vi "Begin.vi"() -> (0 "error out":errorcluster)   [LabVIEW 2013]
doc: "Called before other user functions, this VI is expected to open initial I/O refnums, load in file data, and do all program initialization. Notice that the <B>error out</B> terminal is simply used for data flow. Wiring it to other structures or subVIs ensures that this VI runs first."
uses:
  <vilib>/Rock Robotics/WPI/DriverStation/WPI_DriverStationRobotMode2.ctl
  <vilib>/Rock Robotics/WPI/Joystick/WPI_JoystickDeviceEnum.ctl
  <vilib>/Rock Robotics/SystemInterfaces/DIO/FPGA_DIOPWMChannel.ctl
  <vilib>/Rock Robotics/SystemInterfaces/AI/FPGA_AIChannel.ctl
  <vilib>/Rock Robotics/SystemInterfaces/DIO/FPGA_DIOChannel.ctl
  <vilib>/Rock Robotics/WPI/Encoder/WPI_EncoderType.ctl
  Robot Global Data.vi
  <vilib>/Rock Robotics/WPI/MotorControl/WPI_MotorControlOpen Talon.vi
  <vilib>/Rock Robotics/WPI/Counter/WPI_CounterDigitalInputToDigitalSource.vi
  <vilib>/Utility/file.llb/Read From Spreadsheet File (DBL).vi
  Globals/Auto.vi
  Globals/Homes.vi
  <vilib>/Rock Robotics/WPI/Camera/WPI_CameraWhite Balance Values.ctl
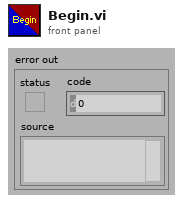
[diagram p1: front panel]
types:
  T1 = typedef "FPGA_DIOPWMChannel.ctl" = enum8{"PWM 1", "PWM 2", "PWM 3", "PWM 4", "PWM 5", "PWM 6", "PWM 7", "PWM 8", "PWM 9", "PWM 10", "Invalid"}
  T2 = typedef "FPGA_AIChannel.ctl" = enum8{"AI 1", "AI 2", "AI 3", "AI 4", "AI 5", "AI 6", "AI 7", "AI 8", "Invalid"}
  T3 = typedef "FPGA_DIOChannel.ctl" = enum8{"DIO 1", "DIO 2", "DIO 3", "DIO 4", "DIO 5", "DIO 6", "DIO 7", "DIO 8", "DIO 9", "DIO 10", "DIO 11", "DIO 12", "DIO 13", "DIO 14", "Invalid"}
  T4 = typedef "WPI_EncoderType.ctl" = enum16{"1x", "2x", "4x"}
  T5 = typedef "WPI_JoystickDeviceEnum.ctl" = enum16{"USB 1", "USB 2", "USB 3", "USB 4", "Kinect 1", "Kinect 2"}
  T6 = typedef "WPI_DriverStationRobotMode2.ctl" = enum16{"Autonomous Disabled", "Autonomous Enabled", "Teleop Disabled", "Teleop Enabled", "Timeout", "Finish", "Test Disabled", "Test Enabled"}
  T7 = typedef "WPI_JoystickDevRef.ctl" = cluster{"Device":T5}
  T8 = typedef "WPI_MotorControlDeviceRef.ctl" = cluster{"DeviceStatus":errorcluster, "Type":enum16{"PWM", "CAN"}, "PWM":cluster{"Digital Module":T9, "PWM Channel":T1, "DeadBand":T10}, "CAN":cluster{"Device Number":u8, "Control Mode":T11, "Semaphore":T12, "Max Vout":dbl}, "Invert":bool, "TransformRef":T13, "InvTransformRef":T13}
  T9 = typedef "FPGA_TypedefDigitalModule.ctl" = enum16{"Digital Module 1", "Digital Module 2"}
  T10 = typedef "WPI_PWMDeadband.ctl" = cluster{"Name":string, "maxPositivePwm":i32, "minPositivePwm":i32, "centerPwm":i32, "maxNegativePwm":i32, "minNegativePwm":i32, "angularRange":u16}
  T11 = typedef "WPI_CANJaguar_ControlMode.ctl" = enum8{"Percent VBus", "Current", "Speed", "Position", "Voltage"}
  T12 = typedef "Semaphore RefNum" = refnum<k1>
  T13 = typedef "WPI_PWMTransform_ConPane.ctl" = refnum<vi>
  T14 = typedef "WPI_CameraWhite Balance Values.ctl" = enum16{"Auto", "Fixed indoor", "Fixed outdoor 1", "Fixed outdoor 2", "Fixed fluorescent 1", "Fixed fluorescent 2", "Hold current"}
  T15 = typedef "WPI_CameraDevRef.ctl" = cluster{"Camera Address":string, "CameraStatus":errorcluster, "Acquire Image Notifier":refnum<notifier>}
  T16 = typedef "WPI_AnalogChannelDevRef.ctl" = cluster{"DevStatus":errorcluster, "Analog Module":T17, "Analog Channel":T2}
  T17 = typedef "FPGA_TypedefAnalogModule.ctl" = enum16{"Analog Module 1", "Analog Module 2"}
  T18 = typedef "WPI_DigitalInputDevRef.ctl" = cluster{"DevStatus":errorcluster, "DIO Channel":T3, "Digital Module":T9}
  T19 = typedef "FPGA_CounterEncoderSourceConvertionLVSourceType.ctl" = cluster{"DevStatus":errorcluster, "AnalogTriggerMode?":bool, "DigitalMode":cluster{"Digital Module":T9, "DIO Channel":T20}, "AnalogTriggerMode":cluster{"AnalogTriggerIndex":T21, "OutputType":T22}}
  T20 = typedef "FPGA_DIODigitalSourceChannel.ctl" = enum8{"DIO 1", "DIO 2", "DIO 3", "DIO 4", "DIO 5", "DIO 6", "DIO 7", "DIO 8", "DIO 9", "DIO 10", "DIO 11", "DIO 12", "DIO 13", "DIO 14", "Disabled"}
  T21 = typedef "FPGA_AnalogTriggerIndex.ctl" = enum8{"Trig 0", "Trig 1", "Trig 2", "Trig 3", "Trig 4", "Trig 5", "Trig 6", "Trig 7", "Invalid"}
  T22 = typedef "FPGA_AnalogTriggerOutType.ctl" = enum16{"InWindow", "TriggerState", "Rising", "Falling"}
  T23 = typedef "WPI_EncoderDevRef.ctl" = cluster{"DevStatus":errorcluster, "EncoderIndex":T24, "CounterIndex":T25, "DistancePerCount":dbl, "Decoding Type":T4}
  T24 = typedef "FPGA_EncoderIdx.ctl" = enum8{"Enc 0", "Enc 1", "Enc 2", "Enc 3", "Invalid"}
  T25 = typedef "FPGA_CounterCtrSystemIndex.ctl" = enum8{"Ctr 0", "Ctr 1", "Ctr 2", "Ctr 3", "Ctr 4", "Ctr 5", "Ctr 6", "Ctr 7", "Invalid"}
  T26 = typedef "WPI_DigitalOutputDevRef.ctl" = cluster{"Digital Module":T9, "DIO Channel":T3, "DevStatus":errorcluster}
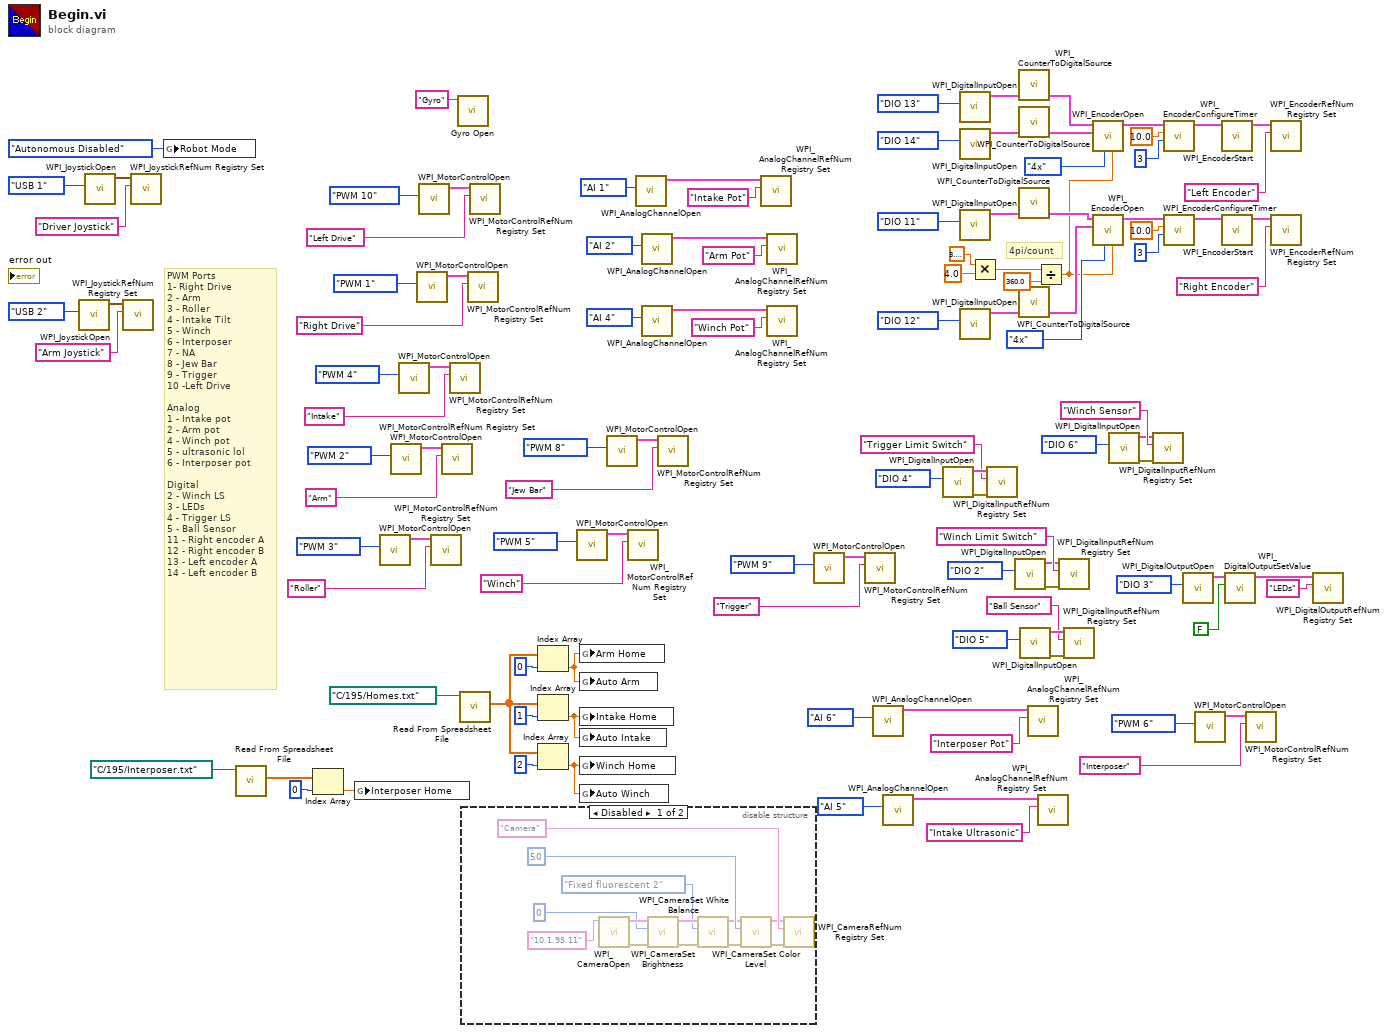
[diagram p0: block diagram]
diagram:
  # "4pi/count"
  # "PWM Ports\n1- Right Drive\n2 - Arm\n3 - Roller\n4 - Intake Tilt \n5 - Winch\n6 - Interposer \n7 - NA\n8 - Jew Bar\n9 - Trigger\n10 -Left Drive\n\nAnalog\n1 - Intake pot\n2 - Arm pot\n4 - Winch pot\n5 - ultrasonic lol\n6 - Interposer pot\n\nDigital \n2 - Winch LS\n3 - LEDs\n4 - Trigger LS\n5 - Ball Sensor\n11 - Right encoder A\n12 - Right encoder B\n13 - Left encoder A\n14 - Left encoder B"
  n1 = call <vilib>:"WPI_JoystickOpen.vi"("JoystickDevice"=WPI_JoystickDeviceEnum."USB 2") -> ("JoystickDevRef"=w109:T7)  [unwired: 10 in]
  n2 = call <vilib>:"WPI_JoystickOpen.vi"("JoystickDevice"=WPI_JoystickDeviceEnum."USB 1") -> ("JoystickDevRef"=w112:T7)  [unwired: 10 in]
  n3 = call <vilib>:"WPI_JoystickRefNum Registry Set.vi"("refnum name"="Arm Joystick", "JoystickDevRef"=w109) -> ()  [unwired: 8 in, 2 out]
  n4 = call <vilib>:"WPI_JoystickRefNum Registry Set.vi"("refnum name"="Driver Joystick", "JoystickDevRef"=w112) -> ()  [unwired: 8 in, 2 out]
  n5 = global write "Robot Global Data.vi" "Robot Mode"(WPI_DriverStationRobotMode2."Autonomous Disabled" ("Robot Mode")) -> ()
  n6 = call-poly <vilib>:"Read From Spreadsheet File.vi"("file path (dialog if empty)"=path "C:/195/Interposer.txt" ("file path (use dialog)")) -> ("first row"=w2:dbl[])  [unwired: 6 in, 4 out]
  n7 = Index Array(array=w2, index=0) -> (element=w1:dbl)
  n8 = global write "Homes.vi" "Interposer Home"(w1) -> ()
  n9 = call-poly <vilib>:"WPI_MotorControlOpen.vi"("PWM Channel"=FPGA_DIOPWMChannel."PWM 3") -> ("MotorControlDeviceRef"=w95:T8)  [unwired: 9 in, 1 out]
  n10 = call-poly <vilib>:"WPI_MotorControlOpen.vi"("PWM Channel"=FPGA_DIOPWMChannel."PWM 2") -> ("MotorControlDeviceRef"=w98:T8)  [unwired: 9 in, 1 out]
  n11 = call-poly <vilib>:"WPI_MotorControlOpen.vi"("PWM Channel"=FPGA_DIOPWMChannel."PWM 4") -> ("MotorControlDeviceRef"=w99:T8)  [unwired: 9 in, 1 out]
  n12 = call-poly <vilib>:"WPI_MotorControlOpen.vi"("PWM Channel"=FPGA_DIOPWMChannel."PWM 1") -> ("MotorControlDeviceRef"=w102:T8)  [unwired: 9 in, 1 out]
  n13 = call-poly <vilib>:"WPI_MotorControlOpen.vi"("PWM Channel"=FPGA_DIOPWMChannel."PWM 10") -> ("MotorControlDeviceRef"=w107:T8)  [unwired: 9 in, 1 out]
  n14 = call <vilib>:"WPI_MotorControlRefNum Registry Set.vi"("refnum name"="Roller", "MotorControlDevRef"=w95) -> ()  [unwired: 8 in, 2 out]
  n15 = call <vilib>:"WPI_MotorControlRefNum Registry Set.vi"("refnum name"="Arm", "MotorControlDevRef"=w98) -> ()  [unwired: 8 in, 2 out]
  n16 = call <vilib>:"WPI_MotorControlRefNum Registry Set.vi"("refnum name"="Intake", "MotorControlDevRef"=w99) -> ()  [unwired: 8 in, 2 out]
  n17 = call "Gyro Open.vi"("refnum name"="Gyro") -> ()  [unwired: 10 in, 1 out]
  n18 = call-poly <vilib>:"Read From Spreadsheet File.vi"("file path (dialog if empty)"=path "C:/195/Homes.txt" ("file path (use dialog)")) -> ("first row"=w28:dbl[])  [unwired: 6 in, 4 out]
  n19 = disable-structure shown="Disabled" {
    frame Disabled {
      n20 = call <vilib>:"WPI_CameraOpen.vi"("Camera Address"="10.1.95.11") -> ("error out"=w121:errorcluster, "CameraDevRef"=w126:T15)  [unwired: 1 in, 8 out]
      n21 = call <vilib>:"WPI_CameraSet Brightness.vi"("error in (no error)"=w121, "Brightness"=0, "CameraDevRef"=w126) -> ("error out"=w122:errorcluster, "CameraDevRef Out"=w125:T15)  [unwired: 7 in]
      n22 = call <vilib>:"WPI_CameraSet White Balance.vi"("error in (no error)"=w122, "White Balance"=WPI_CameraWhite_Balance_Values."Fixed fluorescent 2", "CameraDevRef"=w125) -> ("error out"=w117:errorcluster, "CameraDevRef Out"=w115:T15)  [unwired: 7 in]
      n23 = call <vilib>:"WPI_CameraSet Color Level.vi"("error in (no error)"=w117, "Color Level"=50, "CameraDevRef"=w115) -> ("error out"=w118:errorcluster, "CameraDevRef Out"=w119:T15)  [unwired: 7 in]
      n24 = call <vilib>:"WPI_CameraRefNum Registry Set.vi"("error in (no error)"=w118, "refnum name"="Camera", "CameraDevRef"=w119) -> ()  [unwired: 9 out]
    }
    frame Enabled {
    }
  }
  n25 = call <vilib>:"WPI_MotorControlRefNum Registry Set.vi"("refnum name"="Right Drive", "MotorControlDevRef"=w102) -> ()  [unwired: 8 in, 2 out]
  n26 = call <vilib>:"WPI_MotorControlRefNum Registry Set.vi"("refnum name"="Left Drive", "MotorControlDevRef"=w107) -> ()  [unwired: 8 in, 2 out]
  n27 = Index Array(array=w28, index=0) -> (element=w17:dbl)
  n28 = Index Array(array=w28, index=1) -> (element=w15:dbl)
  n29 = Index Array(array=w28, index=2) -> (element=w16:dbl)
  n30 = call-poly <vilib>:"WPI_MotorControlOpen.vi"("PWM Channel"=FPGA_DIOPWMChannel."PWM 5") -> ("MotorControlDeviceRef"=w81:T8)  [unwired: 9 in, 1 out]
  n31 = global write "Homes.vi" "Arm Home"(w17) -> ()
  n32 = global write "Auto.vi" "Auto Arm"(w17) -> ()
  n33 = global write "Homes.vi" "Intake Home"(w15) -> ()
  n34 = global write "Auto.vi" "Auto Intake"(w15) -> ()
  n35 = global write "Homes.vi" "Winch Home"(w16) -> ()
  n36 = global write "Auto.vi" "Auto Winch"(w16) -> ()
  n37 = call-poly <vilib>:"WPI_MotorControlOpen.vi"("PWM Channel"=FPGA_DIOPWMChannel."PWM 8") -> ("MotorControlDeviceRef"=w76:T8)  [unwired: 9 in, 1 out]
  n38 = call <vilib>:"WPI_MotorControlRefNum Registry Set.vi"("refnum name"="Winch", "MotorControlDevRef"=w81) -> ()  [unwired: 8 in, 2 out]
  n39 = call <vilib>:"WPI_AnalogChannelOpen.vi"("Analog Channel"=FPGA_AIChannel."AI 1") -> ("AIDeviceRef"=w92:T16)  [unwired: 9 in, 1 out]
  n40 = call <vilib>:"WPI_AnalogChannelOpen.vi"("Analog Channel"=FPGA_AIChannel."AI 2") -> ("AIDeviceRef"=w87:T16)  [unwired: 9 in, 1 out]
  n41 = call <vilib>:"WPI_AnalogChannelOpen.vi"("Analog Channel"=FPGA_AIChannel."AI 4") -> ("AIDeviceRef"=w86:T16)  [unwired: 9 in, 1 out]
  n42 = call <vilib>:"WPI_MotorControlRefNum Registry Set.vi"("refnum name"="Jew Bar", "MotorControlDevRef"=w76) -> ()  [unwired: 8 in, 2 out]
  n43 = call <vilib>:"WPI_AnalogChannelRefNum Registry Set.vi"("refnum name"="Intake Pot", "AIDeviceRef"=w92) -> ()  [unwired: 8 in, 2 out]
  n44 = call <vilib>:"WPI_AnalogChannelRefNum Registry Set.vi"("refnum name"="Arm Pot", "AIDeviceRef"=w87) -> ()  [unwired: 8 in, 2 out]
  n45 = call <vilib>:"WPI_AnalogChannelRefNum Registry Set.vi"("refnum name"="Winch Pot", "AIDeviceRef"=w86) -> ()  [unwired: 8 in, 2 out]
  n46 = call-poly <vilib>:"WPI_MotorControlOpen.vi"("PWM Channel"=FPGA_DIOPWMChannel."PWM 9") -> ("MotorControlDeviceRef"=w71:T8)  [unwired: 9 in, 1 out]
  n47 = call <vilib>:"WPI_MotorControlRefNum Registry Set.vi"("refnum name"="Trigger", "MotorControlDevRef"=w71) -> ()  [unwired: 8 in, 2 out]
  n48 = call <vilib>:"WPI_AnalogChannelOpen.vi"("Analog Channel"=FPGA_AIChannel."AI 6") -> ("AIDeviceRef"=w8:T16)  [unwired: 9 in, 1 out]
  n49 = call <vilib>:"WPI_AnalogChannelOpen.vi"("Analog Channel"=FPGA_AIChannel."AI 5") -> ("AIDeviceRef"=w27:T16)  [unwired: 9 in, 1 out]
  n50 = call <vilib>:"WPI_DigitalInputOpen.vi"("DIO Channel"=FPGA_DIOChannel."DIO 4") -> ("error out"=w79:errorcluster, "DigitalInputDevRef"=w78:T18)  [unwired: 9 in]
  n51 = call <vilib>:"WPI_DigitalInputOpen.vi"("DIO Channel"=FPGA_DIOChannel."DIO 13") -> ("DigitalInputDevRef"=w47:T18)  [unwired: 9 in, 1 out]
  n52 = call <vilib>:"WPI_DigitalInputOpen.vi"("DIO Channel"=FPGA_DIOChannel."DIO 14") -> ("DigitalInputDevRef"=w46:T18)  [unwired: 9 in, 1 out]
  n53 = call <vilib>:"WPI_DigitalInputOpen.vi"("DIO Channel"=FPGA_DIOChannel."DIO 11") -> ("DigitalInputDevRef"=w45:T18)  [unwired: 9 in, 1 out]
  n54 = call <vilib>:"WPI_DigitalInputOpen.vi"("DIO Channel"=FPGA_DIOChannel."DIO 12") -> ("DigitalInputDevRef"=w44:T18)  [unwired: 9 in, 1 out]
  n55 = Multiply(x=3.141592653589793, y=4.0) -> (x*y=w37:dbl)
  n56 = call <vilib>:"WPI_DigitalInputRefNum Registry Set.vi"("error in (no error)"=w79, "refnum name"="Trigger Limit Switch", "DigitalInputDevRef"=w78) -> ()  [unwired: 7 in, 2 out]
  n57 = call <vilib>:"WPI_DigitalInputOpen.vi"("DIO Channel"=FPGA_DIOChannel."DIO 2") -> ("error out"=w67:errorcluster, "DigitalInputDevRef"=w68:T18)  [unwired: 9 in]
  n58 = call-poly <vilib>:"WPI_CounterToDigitalSource.vi"("DigitalInputDevRef"=w47) -> ("Digital Source"=w58:T19)  [unwired: 6 in]
  n59 = call-poly <vilib>:"WPI_CounterToDigitalSource.vi"("DigitalInputDevRef"=w46) -> ("Digital Source"=w57:T19)  [unwired: 6 in]
  n60 = call-poly <vilib>:"WPI_CounterToDigitalSource.vi"("DigitalInputDevRef"=w45) -> ("Digital Source"=w55:T19)  [unwired: 6 in]
  n61 = call-poly <vilib>:"WPI_CounterToDigitalSource.vi"("DigitalInputDevRef"=w44) -> ("Digital Source"=w56:T19)  [unwired: 6 in]
  n62 = call <vilib>:"WPI_DigitalInputOpen.vi"("DIO Channel"=FPGA_DIOChannel."DIO 5") -> ("error out"=w20:errorcluster, "DigitalInputDevRef"=w19:T18)  [unwired: 9 in]
  n63 = call <vilib>:"WPI_AnalogChannelRefNum Registry Set.vi"("refnum name"="Interposer Pot", "AIDeviceRef"=w8) -> ()  [unwired: 8 in, 2 out]
  n64 = Divide(x=w37, y=360.0) -> (x/y=w35:dbl)
  n65 = call <vilib>:"WPI_AnalogChannelRefNum Registry Set.vi"("refnum name"="Intake Ultrasonic", "AIDeviceRef"=w27) -> ()  [unwired: 8 in, 2 out]
  n66 = call <vilib>:"WPI_DigitalInputRefNum Registry Set.vi"("error in (no error)"=w67, "refnum name"="Winch Limit Switch", "DigitalInputDevRef"=w68) -> ()  [unwired: 7 in, 2 out]
  n67 = call <vilib>:"WPI_DigitalInputRefNum Registry Set.vi"("error in (no error)"=w20, "refnum name"="Ball Sensor", "DigitalInputDevRef"=w19) -> ()  [unwired: 7 in, 2 out]
  n68 = call <vilib>:"WPI_EncoderOpen.vi"("DistancePerCount"=w35, "Decoding Type"=WPI_EncoderType."4x", "BSource"=w57, "ASource"=w58) -> ("EncoderDevRef"=w65:T23)  [unwired: 6 in, 1 out]
  n69 = call <vilib>:"WPI_EncoderOpen.vi"("DistancePerCount"=w35, "Decoding Type"=WPI_EncoderType."4x", "BSource"=w56, "ASource"=w55) -> ("EncoderDevRef"=w48:T23)  [unwired: 6 in, 1 out]
  n70 = call <vilib>:"WPI_DigitalInputOpen.vi"("DIO Channel"=FPGA_DIOChannel."DIO 6") -> ("error out"=w12:errorcluster, "DigitalInputDevRef"=w13:T18)  [unwired: 9 in]
  n71 = call <vilib>:"WPI_DigitalInputRefNum Registry Set.vi"("error in (no error)"=w12, "refnum name"="Winch Sensor", "DigitalInputDevRef"=w13) -> ()  [unwired: 7 in, 2 out]
  n72 = call <vilib>:"WPI_EncoderConfigureTimer.vi"("Number Samples to Average"=u8 3, "Minimum Rate"=10.0, "EncoderDevRef"=w65) -> ("EncoderDevRef"=w64:T23)  [unwired: 7 in, 1 out]
  n73 = call <vilib>:"WPI_EncoderConfigureTimer.vi"("Number Samples to Average"=u8 3, "Minimum Rate"=10.0, "EncoderDevRef"=w48) -> ("EncoderDevRef"=w49:T23)  [unwired: 7 in, 1 out]
  n74 = call <vilib>:"WPI_DigitalOutputOpen.vi"("DIO Channel"=FPGA_DIOChannel."DIO 3") -> ("DigitalOutputDevRef"=w24:T26)  [unwired: 9 in, 1 out]
  n75 = call-poly <vilib>:"WPI_MotorControlOpen.vi"("PWM Channel"=FPGA_DIOPWMChannel."PWM 6") -> ("MotorControlDeviceRef"=w5:T8)  [unwired: 9 in, 1 out]
  n76 = call <vilib>:"WPI_EncoderStart.vi"("EncoderDevRef"=w64) -> ("EncoderDevRef"=w63:T23)  [unwired: 9 in, 1 out]
  n77 = call <vilib>:"WPI_EncoderStart.vi"("EncoderDevRef"=w49) -> ("EncoderDevRef"=w50:T23)  [unwired: 9 in, 1 out]
  n78 = call <vilib>:"WPI_DigitalOutputSetValue.vi"("Value"=FALSE, "DigitalOutputDevRef"=w24) -> ("DigitalOutputDevRef"=w23:T26)  [unwired: 8 in, 1 out]
  n79 = call <vilib>:"WPI_MotorControlRefNum Registry Set.vi"("refnum name"="Interposer", "MotorControlDevRef"=w5) -> ()  [unwired: 8 in, 2 out]
  n80 = call <vilib>:"WPI_EncoderRefNum Registry Set.vi"("refnum name"="Left Encoder", "EncoderDevRef"=w63) -> ()  [unwired: 8 in, 2 out]
  n81 = call <vilib>:"WPI_EncoderRefNum Registry Set.vi"("refnum name"="Right Encoder", "EncoderDevRef"=w50) -> ()  [unwired: 8 in, 2 out]
  n82 = call <vilib>:"WPI_DigitalOutputRefNum Registry Set.vi"("refnum name"="LEDs", "DigitalOutputDevRef"=w23) -> ()  [unwired: 8 in, 2 out]
